vi "WPI_Gyro_ADXRS453_BitArrayToSPI.vi"(11 "32-bit Array in":bool[](array[boolean])) -> (3 "SPI Byte Array (MSB first)":u8[](array[numeric]))   [LabVIEW 2015, in "FRC Gyro and Accel.lvlib"]
uses:
  FRC Gyro and Accel.lvlib
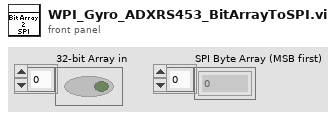
[diagram p1: front panel]
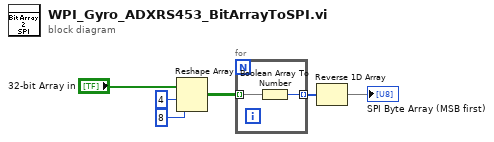
[diagram p0: block diagram]
diagram:
  n1 = Reshape Array("32-bit Array in", 4 ("dimension size"), 8 ("dimension size")) -> (w2:bool[][])
  n2 = for {
    tunnel: w2 -> [w8] mode=indexing
    tunnel: [w7] -> w3 mode=indexing
    n3 = Boolean Array To Number(Boolean array=w8) -> (number=w7:u8)
  }
  n4 = Reverse 1D Array(array=w3) -> (reversed array=→"SPI Byte Array (MSB first)":u8[])
